vi "GetParam.vi"(8 "error in (no error)":errorcluster caption="entrée d'erreur (pas d'erreur)", 11 "Fbeta_Score.lvclass":refnum<class "Fbeta_Score.lvclass">) -> (0 "error out":errorcluster caption="sortie d'erreur", 2 "fbeta_score":T1={"beta"=0.0, "labels"=[], "pos_label"={"dtype_pos_label"="int", "pos_label"="1"}, "average"="binary", "sample_weight"=[], "zero_division"={"dtype_zero_division"="str", "zero_division"="warn"}}, 3 "Fbeta_Score.lvclass":refnum<class "Fbeta_Score.lvclass">)   [LabVIEW 2020, in "Fbeta_Score.lvclass"]
doc: "Get Parameters"
uses:
  Fbeta_Score.lvclass
  Fbeta_Score.lvclass/Fbeta_Score.ctl
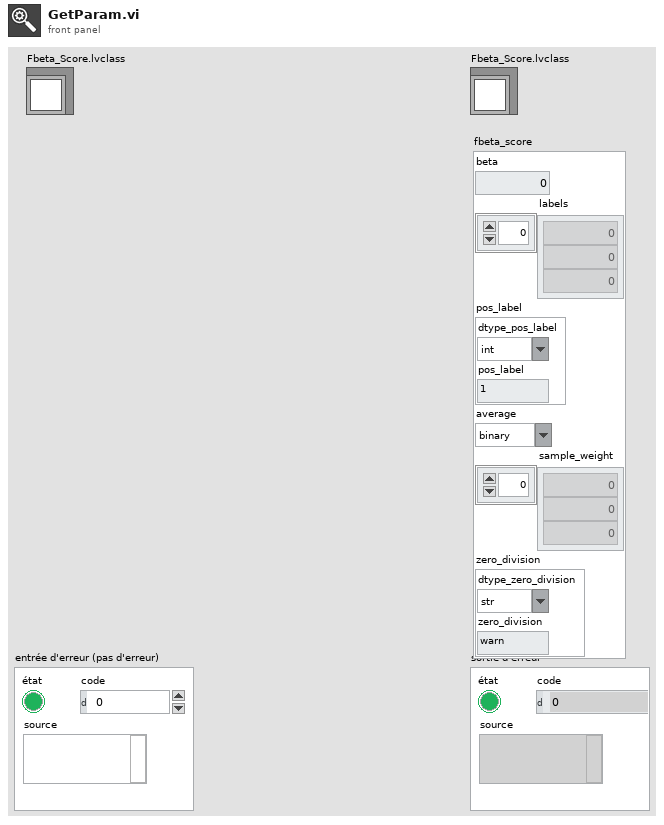
[diagram p1: front panel]
types:
  T1 = cluster{"beta":dbl, "labels":i32[], "pos_label":cluster{"dtype_pos_label":string, "pos_label":string}, "average":string, "sample_weight":dbl[], "zero_division":cluster{"dtype_zero_division":string, "zero_division":string}}
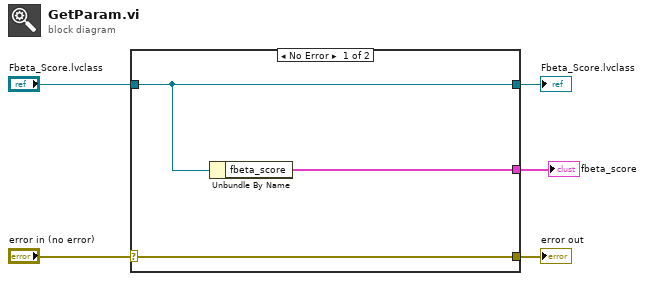
[diagram p0: block diagram]
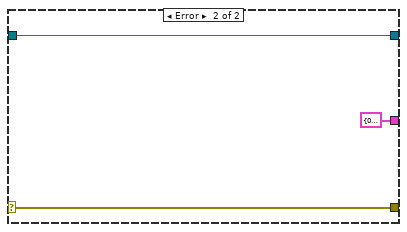
[diagram p2: hidden frame]
diagram:
  n1 = case shown="No Error" "error in (no error)" {
    selector: "error in (no error)" -> [w8 w10]
    tunnel: [w8 w10] -> w4
    tunnel: [w7 w11] -> w2
    tunnel: "Fbeta_Score.lvclass" -> [w7 w11]
    tunnel: [w6 T1 {"beta"=0.0, "labels"=[], "pos_label"={"dtype_pos_label"="", "pos_label"=""}, "average"="", "sample_weight"=[], "zero_division"={"dtype_zero_division"="", "zero_division"=""}} ("fbeta_score")] -> w1
    frame No Error {
      n2 = Unbundle By Name(w7) -> ("fbeta_score"=w6:T1)
    }
    frame Error {
    }
  }
  "error out" <- w4
  "Fbeta_Score.lvclass" <- w2
  "fbeta_score" <- w1
